vi "KeyInCounterPosition V1.00.vi"() -> (1 "Counter Position output":dbl=950.0 min=0.0 max=2600.0 format="%.3f", 2 "Stepper Position":i32)   [LabVIEW 2020]
uses:
  Globals and TypeDefs/Global Varibal Control.vi
panel:
  in  "?":bool
  in  "Counter Position":dbl=7000.0 min=0.0 max=26000.0 format="%.3f"
  # "Please input your own counter position,\nand then click \"OK\" button."
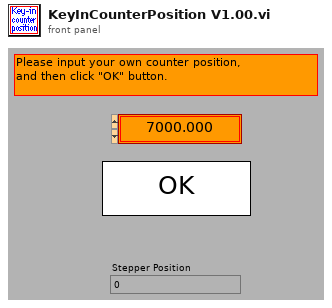
[diagram p1: front panel]
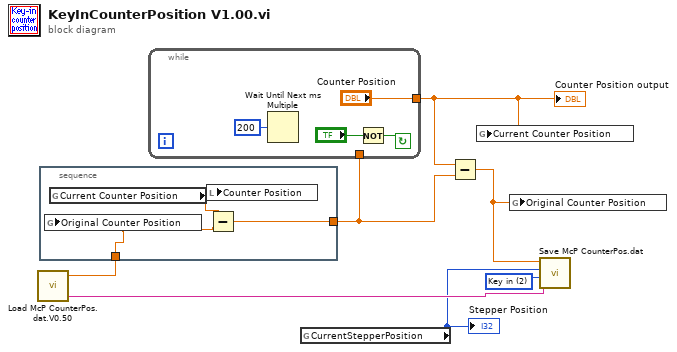
[diagram p0: block diagram]
diagram:
  w6 = u16 2 items=["Moving", "Calibration", "Key in", "Initialization"] ("Set Method")
  n1 = call "Load McP CounterPos.dat.V0.50.vi"() -> ("Counter Position"=w2:dbl, "Last Calibration Date"=w7:string)  [unwired: 1 in, 1 out]
  n2 = stacked-sequence {
    tunnel: [w9] -> w3
    tunnel: w2 -> [w8]
    frame #0 {
      n3 = global write "Global Varibal Control.vi" "Original Counter Position"(w8) -> ()
      n4 = global read "Global Varibal Control.vi" "Current Counter Position"() -> (w10:dbl)
      n5 = local write "Counter Position"(w10) -> ()
      n6 = Subtract(x=w10, y=w8) -> (x-y=w9:dbl)
    }
  }
  n7 = while {
    tunnel: w3 -> [_]
    tunnel: ["Counter Position"] -> w4
    stop <- w14 continue-if-true
    n8 = Wait Until Next ms Multiple(millisecond multiple=u32 200) -> ()  [unwired: 1 out]
    n9 = Not(x="?") -> (.not. x?=w14:bool)
  }
  "Counter Position output" <- w4
  n10 = global read "Global Varibal Control.vi" "CurrentStepperPosition"() -> (w5:i32)
  "Stepper Position" <- w5
  n11 = Subtract(x=w4, y=w3) -> (x-y=w1:dbl)
  n12 = global write "Global Varibal Control.vi" "Current Counter Position"(w4) -> ()
  n13 = global write "Global Varibal Control.vi" "Original Counter Position"(w1) -> ()
  n14 = call "Save McP CounterPos.dat.vi"("Last Calibration Date"=w7, "Set Method"=w6, "McP Stepper Position"=w5, "McP Counter Position"=w1) -> ()  [unwired: 2 in, 1 out]
